vi "GitHub API_List Public Repositories.vi"() -> ()   [LabVIEW 2013]
uses:
  <vilib>/httpClient/LabVIEWHTTPClient.lvlib
  <vilib>/addons/_JKI.lib/Serialization/JSON/JKI JSON Serialization.lvlib
panel:
  out "Public Repositories":cluster{"name":string, "html_url":string}[](array[cluster])
  out "body":string
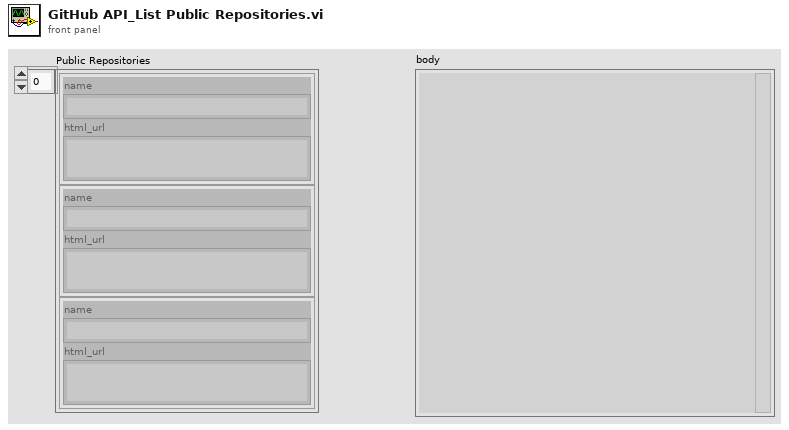
[diagram p1: front panel]
types:
  T1 = typedef "LabVIEWHTTPClient.lvlib/ClientHandle.ctl" = refnum<k1>
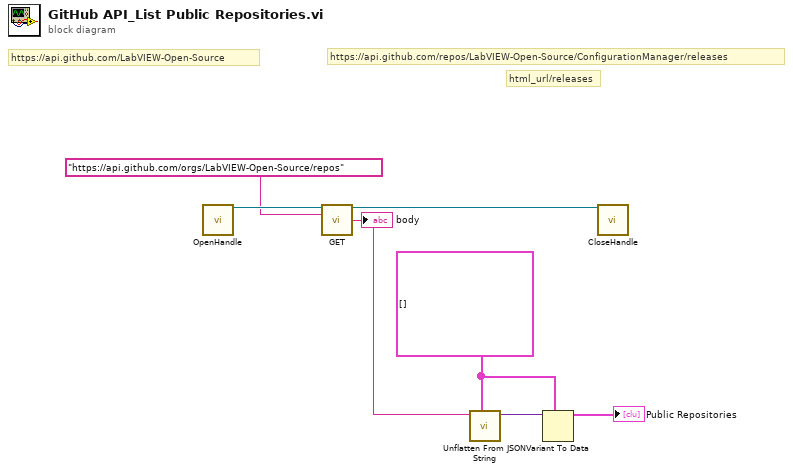
[diagram p0: block diagram]
diagram:
  w1 = cluster{"name":string, "html_url":string}[] []
  # "https://api.github.com/repos/LabVIEW-Open-Source/ConfigurationManager/releases"
  # "html_url/releases"
  # "https://api.github.com/LabVIEW-Open-Source"
  n1 = call <vilib>:"OpenHandle.vi"() -> ("client handle out"=w7:T1)  [unwired: 14 in, 1 out]
  n2 = call <vilib>:"GET.vi"("client handle"=w7, "url"="https://api.github.com/orgs/LabVIEW-Open-Source/repos") -> ("client handle out"=w5:T1, "body"=w4:string)  [unwired: 10 in, 2 out]
  "body" <- w4
  n3 = call <vilib>:"Unflatten From JSON String.vi"("Type and Defaults"=w1, "JSON String"=w4) -> ("Variant"=w3:variant)  [unwired: 8 in, 1 out]
  n4 = Variant To Data(type=w1, Variant=w3) -> (data=→"Public Repositories":cluster{"name":string, "html_url":string}[])  [unwired: 1 in, 1 out]
  n5 = call <vilib>:"CloseHandle.vi"("client handle"=w5) -> ()  [unwired: 14 in, 1 out]
